vi "DisplayLogic_DrawRectangle.vi"(0 "Player":u8, 1 "ActivePixel":cluster{"h_pixel":i16, "v_pixel":i16}, 4 "RectanglePosition":T1) -> (16 "PixelData":bool[](array[boolean]))   [LabVIEW 2018]
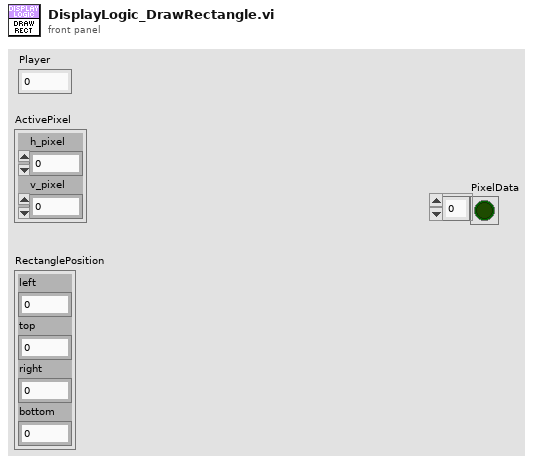
[diagram p1: front panel]
types:
  T1 = cluster{"left":i16, "top":i16, "right":i16, "bottom":i16}
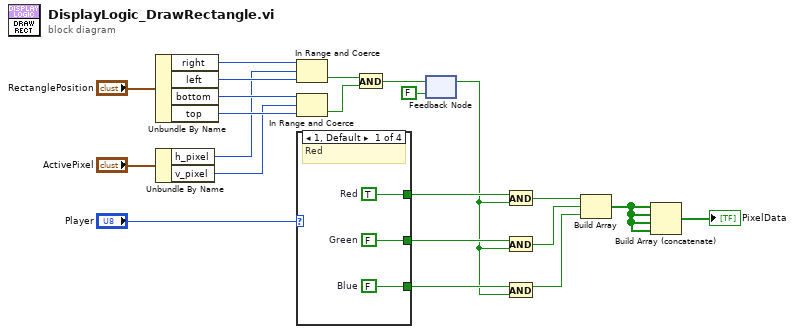
[diagram p0: block diagram]
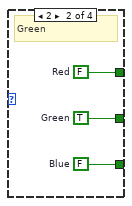
[diagram p2: hidden frame]
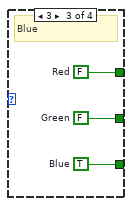
[diagram p3: hidden frame]
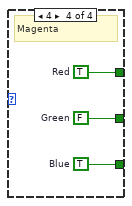
[diagram p4: hidden frame]
diagram:
  n1 = Unbundle By Name("RectanglePosition") -> ("right"=w21:i16, "left"=w20:i16, "bottom"=w19:i16, "top"=w18:i16)
  n2 = Unbundle By Name("ActivePixel") -> ("h_pixel"=w14:i16, "v_pixel"=w13:i16)
  n3 = In Range and Coerce(upper limit=w21, x=w14, lower limit=w20) -> (In Range?=w17:bool)  [unwired: 1 out]
  n4 = In Range and Coerce(upper limit=w19, x=w13, lower limit=w18) -> (In Range?=w16:bool)  [unwired: 1 out]
  n5 = case shown="1, Default" "Player" {
    tunnel: [w25 w28 w31 w34] -> w10
    tunnel: [w24 w27 w30 w33] -> w9
    tunnel: [w23 w26 w29 w32] -> w8
    frame 1, Default {
      w23 = FALSE  # Blue
      w24 = FALSE  # Green
      w25 = TRUE  # Red
      # "Red"
    }
    frame 2 {
      w26 = FALSE  # Blue
      w27 = TRUE  # Green
      w28 = FALSE  # Red
      # "Green"
    }
    frame 3 {
      w29 = TRUE  # Blue
      w30 = FALSE  # Green
      w31 = FALSE  # Red
      # "Blue"
    }
    frame 4 {
      w32 = TRUE  # Blue
      w33 = FALSE  # Green
      w34 = TRUE  # Red
      # "Magenta"
    }
  }
  n6 = And(x=w17, y=w16) -> (x .and. y?=w3:bool)
  n7 = feedback-in #1(w3) -> ()
  n8 = feedback #1(FALSE) -> (w2:bool)
  n9 = And(x=w10, y=w2) -> (x .and. y?=w6:bool)
  n10 = And(x=w9, y=w2) -> (x .and. y?=w5:bool)
  n11 = And(x=w8, y=w2) -> (x .and. y?=w4:bool)
  n12 = Build Array(w6, w5, w4) -> (w7:bool[])
  n13 = Build Array (concatenate)(w7, w7, w7, w7) -> (→"PixelData":bool[])
